vi "StructToString.vi"(8 "error in (no error)":errorcluster, 9 "byte order":T3(ring)=enum."native, host order", 10 "Element and Padding Info":T1, 11 "Data as Unsigned Byte Array (with padding)":u8[](array[numeric])) -> (0 "error out":errorcluster, 1 "byte order (0:big-endian, network order) 2":T3(ring)=enum."native, host order", 2 "Size Included (Always F)":bool, 3 "Data As String for Unflatten Function":string)   [LabVIEW 2013]
doc: "This functions takes a byte array returned from a Call Library Function Node. The byte array is essentially the data at some memory space and may include \"padding\" bytes depending on the host and any #pragma packing directives used in the DLL. \n\nThis function is intended to be used after the original LabVIEW cluster has been evaluated and passed into the CLFN by the \"ClusterToCStructByteArray.vi\" which will provide the \"Data Mask\" values this function reqiures.\n\nUse the magic LV-native \"Unflatten From String\" to take the output of this VI and format as the original cluster (could be a type-def, etc.)"
uses:
  TypeDefs/ctl_ElementAndPaddingInfo.ctl
  TypeDefs/ctl_DataElementInfo.ctl
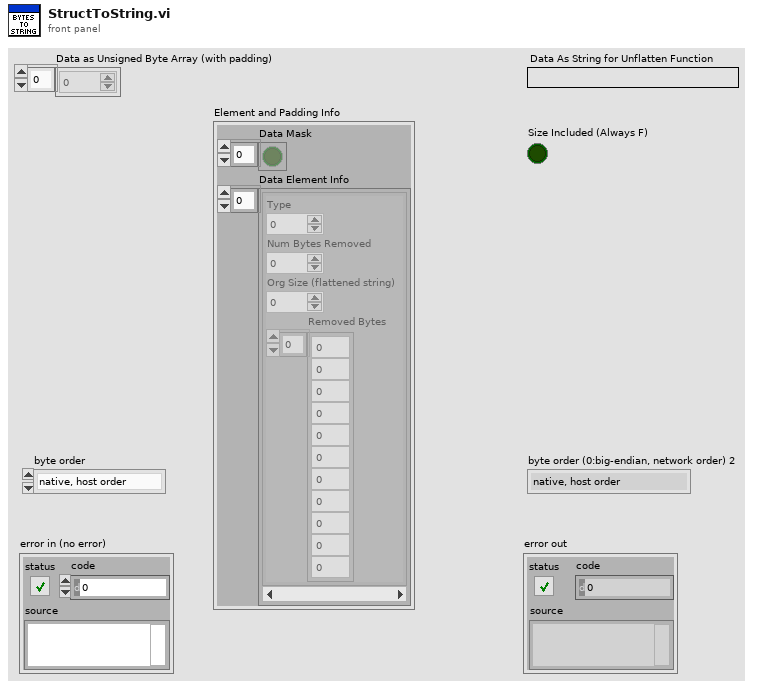
[diagram p1: front panel]
types:
  T1 = typedef "ctl_ElementAndPaddingInfo.ctl" = cluster{"Data Mask":bool[], "Data Element Info":T2[]}
  T2 = typedef "ctl_DataElementInfo.ctl" = cluster{"Type":u16, "Num Bytes Removed":u16, "Org Size (flattened string)":i32, "Removed Bytes":u8[]}
  T3 = enum16{"big-endian, network order", "native, host order", "little-endian"}
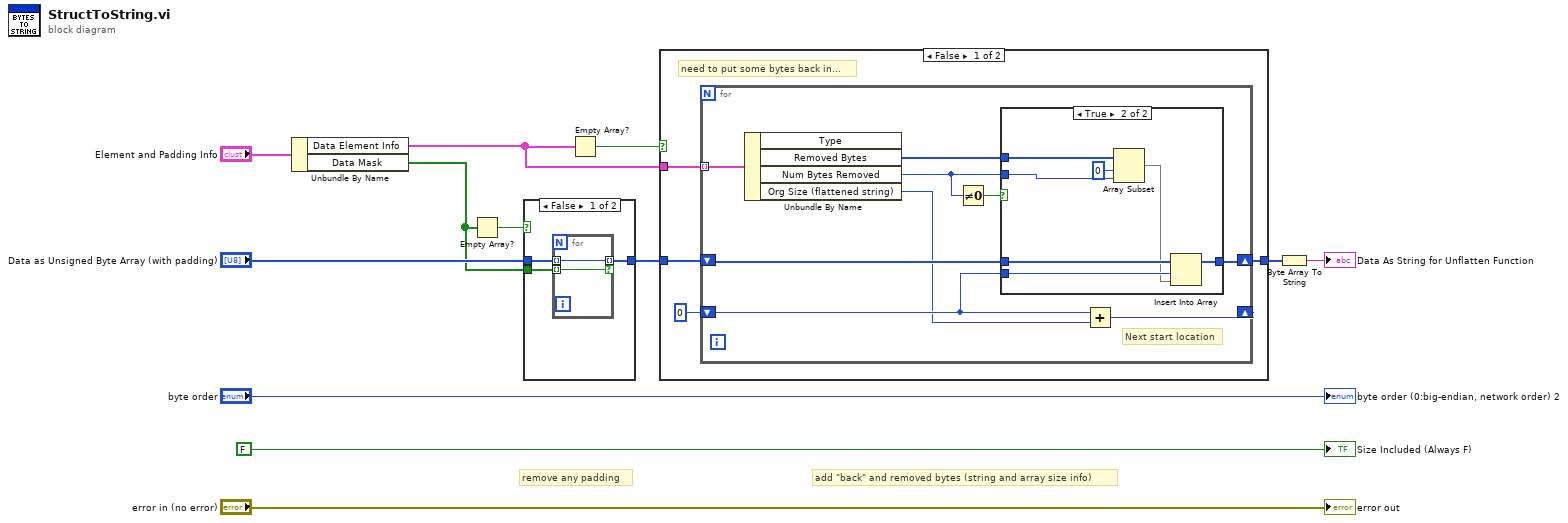
[diagram p0: block diagram]
diagram:
  # "add \"back\" and removed bytes (string and array size info)"
  # "remove any padding"
  n1 = Unbundle By Name("Element and Padding Info") -> ("Data Element Info"=w4:T2[], "Data Mask"=w5:bool[])
  n2 = Empty Array?(array=w5) -> (empty?=w2:bool)
  n3 = case shown="False" w2 {
    tunnel: "Data as Unsigned Byte Array (with padding)" -> [w15 w18]
    tunnel: [w14 w18] -> w7
    tunnel: w5 -> [w13 _]
    frame False {
      n4 = for {
        tunnel: w13 -> [w17] mode=indexing
        tunnel: w15 -> [w16] mode=indexing
        tunnel: [w16] -> w14 mode=indexing if=w17
      }
    }
    frame True {
      # "no mask or no bytes added"
    }
  }
  n5 = Empty Array?(array=w4) -> (empty?=w3:bool)
  n6 = case shown="False" w3 {
    tunnel: w7 -> [w22 w40]
    tunnel: [w21 w40] -> w6
    tunnel: w4 -> [w19 _]
    frame False {
      # "need to put some bytes back in..."
      n7 = for {
        shift-right: [w29] -> w21
        shift-left: w22 -> [w30]
        tunnel: w19 -> [w31] mode=indexing
        shift-right: [w24] -> _
        shift-left: 0 -> [w25]
        # "Next start location"
        n8 = Unbundle By Name(w31) -> ("Removed Bytes"=w26:u8[], "Num Bytes Removed"=w27:u16, "Org Size (flattened string)"=w23:i32)  [unwired: 1 out]
        n9 = Not Equal To 0?(x=w27) -> (x != 0?=w28:bool)
        n10 = case shown="True" w28 {
          tunnel: w30 -> [w32 w39]
          tunnel: [w32 w38] -> w29
          tunnel: w27 -> [_ w36]
          tunnel: w25 -> [_ w35]
          tunnel: w26 -> [_ w33]
          frame False {
          }
          frame True {
            n11 = Array Subset(array=w33, index=0, length=w36) -> (w34:u8[])
            n12 = Insert Into Array(array=w39, index=w35, new element=w34) -> (w38:u8[])
          }
        }
        n13 = Add(x=w25, y=w23) -> (x+y=w24:i32)
      }
    }
    frame True {
      # "nothing to add"
    }
  }
  n14 = Byte Array To String(unsigned byte array=w6) -> (string=→"Data As String for Unflatten Function":string)
  "byte order (0:big-endian, network order) 2" <- "byte order"
  "Size Included (Always F)" <- FALSE ("Size Included (F)")
  "error out" <- "error in (no error)"
